vi "pp2_updateStateInfoTime.vi"(10 "DAQ In":T2, 11 "State In":T3={"Curr  tr"=0, "Curr (ms)"=0, "Cum (ms)"=0, "Run loop diff"=0, "Curr State"=enum."0 Initialization", "Prev State"=enum."0 Initialization", "Sw1"=FALSE, "Tone Gate"=FALSE, "Stim"=FALSE, "Sw2"=FALSE, "Curr code"=0, "Current Trial"={"Trial Type Number"=1, "Trial Type"=enum."GO", "Trial Weight"=100, "Shock (mA)"=0.3, "Duration (ms)"=0.25, "Type"=enum."04 FM Sweep", "Stim P2"=4000.0, "Stim P3"=0.0, "Stim P4"=0.0, "Stim P1"=2000.0}, "Last tone"=0, "Countdown (ms)"=0, "Next Trial"={"Trial Type Number"=1, "Trial Type"=enum."GO", "Trial Weight"=100, "Shock (mA)"=0.3, "Duration (ms)"=0.25, "Type"=enum."04 FM Sweep", "Stim P2"=4000.0, "Stim P3"=0.0, "Stim P4"=0.0, "Stim P1"=2000.0}, "Current DAQ Digital Out"=0} {"Current DAQ Digital Out" format="%b"; "Next Trial"."Shock (mA)" min=-1.0 max=5.0; "Next Trial"."Trial Weight" step=1; "Next Trial"."Duration (ms)" min=0.0 max=1.0; "Next Trial"."Trial Type Number" min=1 max=256 step=1; "Current Trial"."Shock (mA)" min=-1.0 max=5.0; "Current Trial"."Trial Weight" step=1; "Current Trial"."Duration (ms)" min=0.0 max=1.0; "Current Trial"."Trial Type Number" min=1 max=256 step=1; "Curr code" format="%#.6f"}) -> (1 "State timeout":bool, 2 "DAQ Out":T1, 3 "State Out":T3={"Curr  tr"=0, "Curr (ms)"=0, "Cum (ms)"=0, "Run loop diff"=0, "Curr State"=enum."0 Initialization", "Prev State"=enum."0 Initialization", "Sw1"=FALSE, "Tone Gate"=FALSE, "Stim"=FALSE, "Sw2"=FALSE, "Curr code"=0, "Current Trial"={"Trial Type Number"=1, "Trial Type"=enum."GO", "Trial Weight"=100, "Shock (mA)"=0.3, "Duration (ms)"=0.25, "Type"=enum."04 FM Sweep", "Stim P2"=4000.0, "Stim P3"=0.0, "Stim P4"=0.0, "Stim P1"=2000.0}, "Last tone"=0, "Countdown (ms)"=0, "Next Trial"={"Trial Type Number"=1, "Trial Type"=enum."GO", "Trial Weight"=100, "Shock (mA)"=0.3, "Duration (ms)"=0.25, "Type"=enum."04 FM Sweep", "Stim P2"=4000.0, "Stim P3"=0.0, "Stim P4"=0.0, "Stim P1"=2000.0}, "Current DAQ Digital Out"=0} {"Current DAQ Digital Out" format="%b"; "Next Trial"."Shock (mA)" min=-1.0 max=5.0; "Next Trial"."Trial Weight" step=1; "Next Trial"."Duration (ms)" min=0.0 max=1.0; "Next Trial"."Trial Type Number" min=1 max=256 step=1; "Current Trial"."Shock (mA)" min=-1.0 max=5.0; "Current Trial"."Trial Weight" step=1; "Current Trial"."Duration (ms)" min=0.0 max=1.0; "Current Trial"."Trial Type Number" min=1 max=256 step=1; "Curr code" format="%#.6f"}, 4 "Side change":bool, 6 "State change":bool)   [LabVIEW 2013]
uses:
  <vilib>/DAQmx/read.llb/DAQmx Read (Digital 1D Bool NChan 1Samp 1Line).vi
  pp2_State.ctl
  pp2_CTL_StateInfo.ctl
  pp2_TrialType.ctl
  labolabo2/waveforms/WFTypes.ctl
  pp2_Trial.ctl
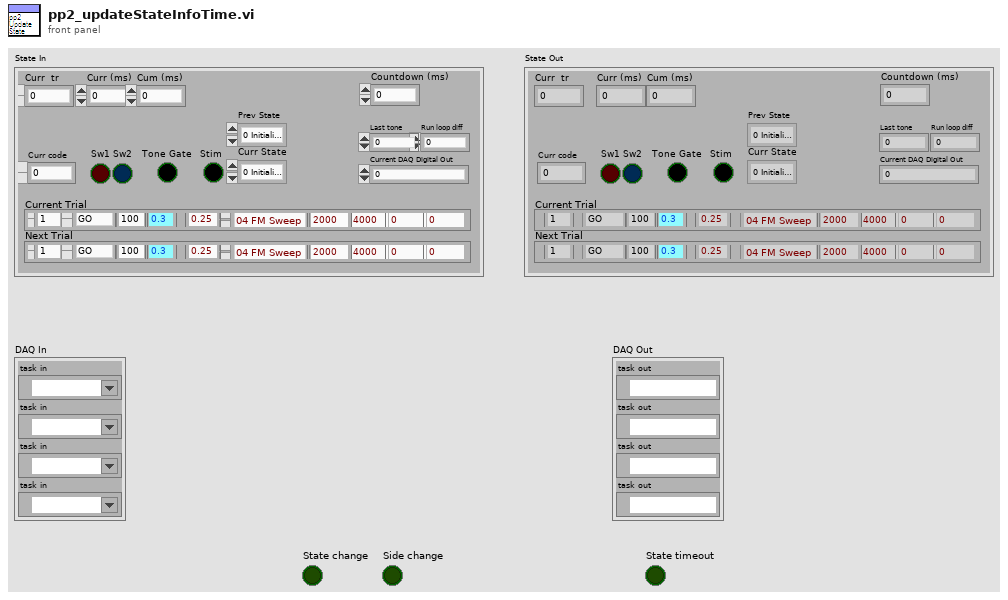
[diagram p1: front panel]
types:
  T1 = cluster{"task out":refnum<k21>, "task out":refnum<k21>, "task out":refnum<k21>, "task out":refnum<k21>}
  T2 = cluster{"task in":refnum<k21>, "task in":refnum<k21>, "task in":refnum<k21>, "task in":refnum<k21>}
  T3 = typedef "pp2_CTL_StateInfo.ctl" = cluster{"Curr  tr":u16, "Curr (ms)":i64, "Cum (ms)":i64, "Run loop diff":i64, "Curr State":T4, "Prev State":T4, "Sw1":bool, "Tone Gate":bool, "Stim":bool, "Sw2":bool, "Curr code":u8, "Current Trial":T5, "Last tone":i64, "Countdown (ms)":i64, "Next Trial":T5, "Current DAQ Digital Out":u16}
  T4 = typedef "pp2_State.ctl" = enum8{"0 Initialization", "1 Habituation", "2 Load Pre", "3 Wait", "4 Pre/Load Trial", "5 GO Trial", "6 GO Jumped", "7 GO Timeout", "8 NOGO Trial", "9 NOGO Jumped", "10 NOGO Timeout", "11 TEST Trial", "12 TEST Jumped", "13 TEST Timeout", "14 Done"}
  T5 = typedef "pp2_Trial.ctl" = cluster{"Trial Type Number":i16, "Trial Type":T6, "Trial Weight":u32, "Shock (mA)":dbl, "Duration (ms)":dbl, "Type":T7, "Stim P2":dbl, "Stim P3":dbl, "Stim P4":dbl, "Stim P1":dbl}
  T6 = typedef "pp2_TrialType.ctl" = enum16{"OFF", "GO", "NOGO", "TEST"}
  T7 = typedef "WFTypes.ctl" = enum16{"00 NULL", "01 DC", "02 Noise", "03 Pure Tone", "04 FM Sweep"}
  T8 = cluster{"task in":refnum<k21>, "task in":refnum<k21>, "task in":refnum<k21>, "task out":refnum<k21>}
  T9 = cluster{"Trial Type Number":i64, "Trial Type":i64, "Trial Weight":i64, "Shock (mA)":dbl, "Duration (ms)":dbl, "Type":i64, "Stim P2":dbl, "Stim P3":dbl, "Stim P4":dbl, "Stim P1":dbl}
  T10 = cluster{"Trial Type Number":bool, "Trial Type":bool, "Trial Weight":bool, "Shock (mA)":bool, "Duration (ms)":bool, "Type":bool, "Stim P2":bool, "Stim P3":bool, "Stim P4":bool, "Stim P1":bool}
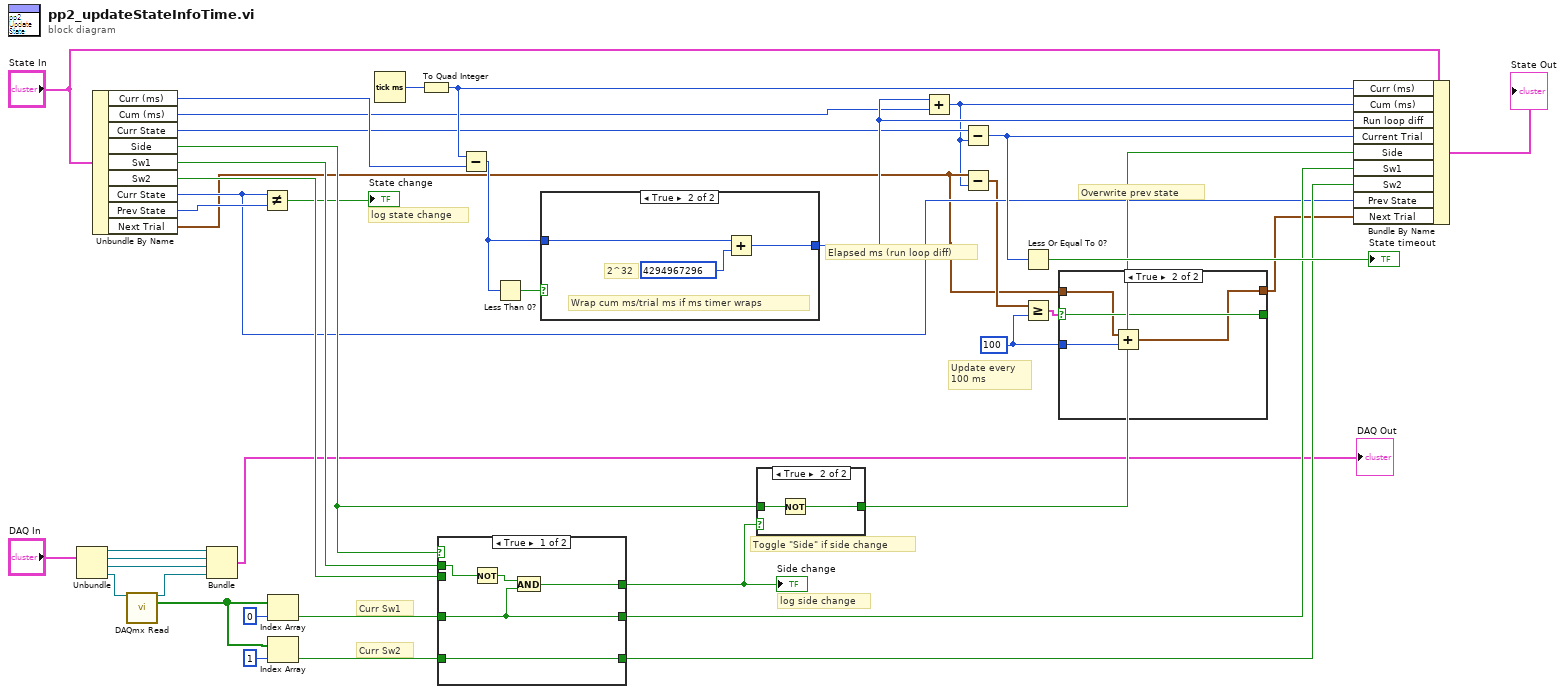
[diagram p0: block diagram]
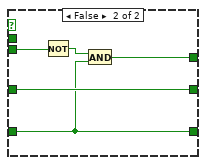
[diagram p4: hidden frame]
diagram:
  w1 = i64 100 ("y")
  # "Update every\n100 ms"
  # "Curr Sw2"
  # "Curr Sw1"
  # "Elapsed ms (run loop diff)"
  # "Overwrite prev state"
  # "log state change"
  # "log side change"
  # "Toggle \"Side\" if side change"
  n1 = Unbundle("DAQ In") -> ("task in"=w15:refnum<k21>, "task in"=w14:refnum<k21>, "task in"=w13:refnum<k21>, "task in"=w28:refnum<k21>)
  n2 = Unbundle By Name("State In") -> ("Curr (ms)"=w35:i64, "Cum (ms)"=w33:i64, "Curr State"=w32:T4, "Side"=w19:bool, "Sw1"=w22:bool, "Sw2"=w21:bool, "Curr State"=w8:T4, "Prev State"=w10:T4, "Next Trial"=w5:T5)
  n3 = call-poly <vilib>:"DAQmx Read.vi"("task/channels in"=w28) -> ("task out"=w12:refnum<k21>, "data"=w25:bool[])  [unwired: 12 in, 1 out]
  n4 = Bundle("task in"=w15, "task in"=w14, "task in"=w13, "task out"=w12) -> (→"DAQ Out":T8)  [unwired: 1 in]
  n5 = Not Equal?(x=w8, y=w10) -> (x != y?=→"State change":bool)
  n6 = Index Array(array=w25, index=0) -> (element=w24:bool)
  n7 = Index Array(array=w25, index=1) -> (element=w23:bool)
  n8 = Tick Count (ms)() -> (millisecond timer value=w41:u32)
  n9 = To Quad Integer(1:w41) -> (0:w36:i64)
  n10 = case shown="True" w19 {
    tunnel: w24 -> [w42 w48]
    tunnel: w23 -> [w44 w47]
    tunnel: w22 -> [w43 _]
    tunnel: w21 -> [_ w51]
    tunnel: [w45 w49] -> w20
    tunnel: [w42 w48] -> w17
    tunnel: [w44 w47] -> w18
    frame True {
      n11 = Not(x=w43) -> (.not. x?=w46:bool)
      n12 = And(x=w46, y=w42) -> (x .and. y?=w45:bool)
    }
    frame False {
      n13 = Not(x=w51) -> (.not. x?=w50:bool)
      n14 = And(x=w50, y=w47) -> (x .and. y?=w49:bool)
    }
  }
  "Side change" <- w20
  n15 = Subtract(x=w36, y=w35) -> (x-y=w39:i64)
  n16 = Less Than 0?(x=w39) -> (x < 0?=w40:bool)
  n17 = case shown="True" w40 {
    tunnel: w39 -> [w52 w54]
    tunnel: [w52 w55] -> w34
    frame False {
    }
    frame True {
      # "Wrap cum ms/trial ms if ms timer wraps"
      # "2^32"
      n18 = Add(x=w54, y=i64 4294967296) -> (x+y=w55:i64)
    }
  }
  n19 = case shown="True" w20 {
    tunnel: w19 -> [w56 w58]
    tunnel: [w56 w57] -> w16
    frame False {
    }
    frame True {
      n20 = Not(x=w58) -> (.not. x?=w57:bool)
    }
  }
  n21 = Add(x=w34, y=w33) -> (x+y=w4:i64)
  n22 = Subtract(x=w32, y=w4) -> (x-y=w30:i64)
  n23 = Subtract(x=w5, y=w4) -> (x-y=w7:T9)
  n24 = Less Or Equal To 0?(x=w30) -> (x <= 0?=→"State timeout":bool)
  n25 = Greater Or Equal?(x=w7, y=w1) -> (x >= y?=w6:T10)
  n26 = case shown="True" w6 {
    selector: w6 -> [w60 w64]
    tunnel: w5 -> [w59 w62]
    tunnel: [w59 w61] -> w3
    tunnel: [w60 w64] -> w2
    tunnel: w1 -> [_ w63]
    frame False {
    }
    frame True {
      n27 = Add(x=w62, y=w63) -> (x+y=w61:T9)
    }
  }
  n28 = Bundle By Name(cluster="State In", "Curr (ms)"=w36, "Cum (ms)"=w4, "Run loop diff"=w34, "Current Trial"=w30, "Side"=w16, "Sw1"=w17, "Sw2"=w18, "Prev State"=w8, "Next Trial"=w3) -> (→"State Out":T3)
